vi "TL show the boat.vi"(2 "GPS":cluster{"X pos":i32, "Y pos":i32, "Heading":dbl}, 3 "Boat array":u32[][](array[numeric]), 4 "Pool array":u32[][](array[numeric])) -> (0 "Invalid Pos?":bool, 1 "Pool out":u32[][](array[numeric]))   [LabVIEW 2014]
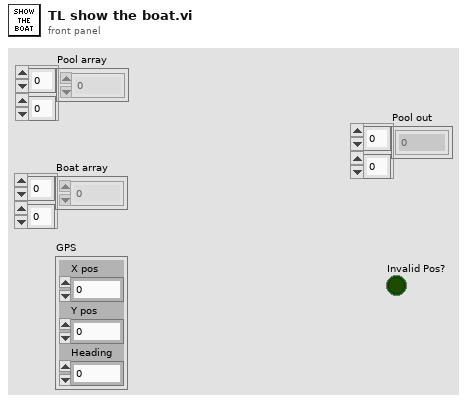
[diagram p1: front panel]
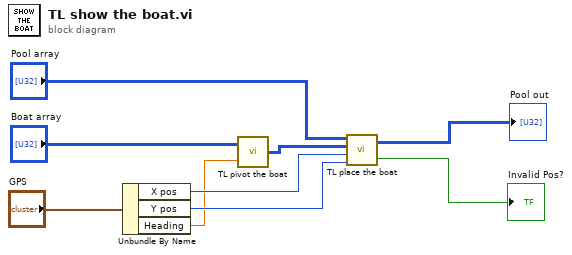
[diagram p0: block diagram]
diagram:
  n1 = Unbundle By Name("GPS") -> ("X pos"=w8:i32, "Y pos"=w7:i32, "Heading"=w6:dbl)
  n2 = call "TL pivot the boat.vi"("Heading"=w6, "Image Pixels (U32)"="Boat array") -> ("Image pixels\nOut"=w9:u32[][])
  n3 = call "TL place the boat.vi"("Y pos"=w7, "X pos"=w8, "Boat image\nPixels (U32)"=w9, "Pool image\nPixels (U32)"="Pool array") -> ("Invalid Pos?"=→"Invalid Pos?":bool, "Pool image\nPixels (U32) out"=→"Pool out":u32[][])
